vi "projector status.vi"(5 "module path":path, 7 "Threshold":dbl format="%#_13g", 8 "error in":errorcluster, 10 "Image IN":T1(plugin-control), 11 "session in":refnum<k35>) -> (0 "error out":errorcluster, 2 "Projector Status":bool, 3 "session out":refnum<k35>)   [LabVIEW 2019, in "Setting Lib.lvlib"]
uses:
  Setting Lib.lvlib
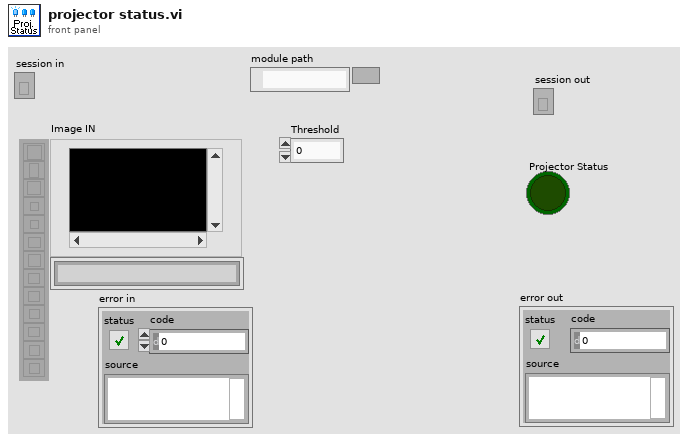
[diagram p1: front panel]
types:
  T1 = typedef "IMAQ Image.ctl" = refnum<image>
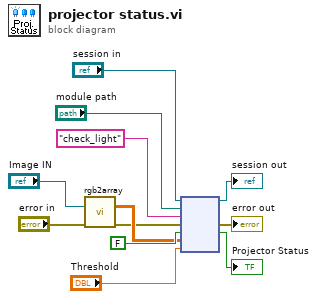
[diagram p0: block diagram]
diagram:
  n1 = call "rgb2array.vi"("Image IN"="Image IN", "error in (no error)"="error in") -> ("output Array"=w8:dbl[][][], "error out"=w1:errorcluster)  [unwired: 12 in]
  n2 = node("session in", "module path", "check_light" ("function name"), w1, FALSE, w8, "Threshold") -> (→"session out":refnum<k35>, →"error out":errorcluster, →"Projector Status":bool)  [unwired: 2 in, 2 out]
